vi "test1-testModuleExitEventAPI.vi"(8 "error in (no error)":errorcluster, 11 "TestCase in":refnum<class "testcase-CSMNonCSMCallerSupportAPI.lvclass">) -> (0 "error out":errorcluster, 3 "TestCase out":refnum<class "testcase-CSMNonCSMCallerSupportAPI.lvclass">)   [LabVIEW 2017, in "testcase-CSMNonCSMCallerSupportAPI.lvclass"]
uses:
  testcase-CSMNonCSMCallerSupportAPI.lvclass
  InternalCluster.ctl
  State_Cluster.ctl
  GlobalVariable_CSMModeData.vi
  <vilib>/addons/_JKI Toolkits/VI Tester/TestCase.llb/TestCase.lvclass
  src/user.lib/_NEVSTOP/Communicable State Machine(CSM)/Communicable State Machine.lvlib
  C:/Program Files (x86)/National Instruments/LabVIEW 2017/vi.lib/addons/_JKI Toolkits/VI Tester/TestCase.llb/TestCase.lvclass
panel:
  out "LoopCount":i32
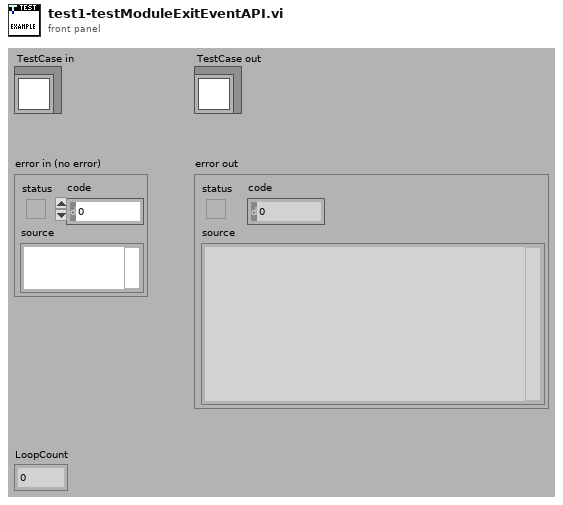
[diagram p1: front panel]
types:
  T1 = typedef "testcase-CSMNonCSMCallerSupportAPI.lvclass/InternalCluster.ctl" = cluster{"Mode":enum16{"Invalid", "Others", "WorkerAgent or Chain"}, "#Nodes":u32}
  T2 = typedef "testcase-CSMNonCSMCallerSupportAPI.lvclass/State_Cluster.ctl" = enum16{"Idle", "Initialize", "PreExit", "Exit"}
  T3 = enum16{"Invalid", "Others", "WorkerAgent or Chain"}
  T4 = typedef "Communicable State Machine.lvlib/_CSM_MODE.ctl" = enum16{"Not Exist", "Stand Alone", "CSM", "Worker", "Worker Agent", "Chain Node", "Chain"}
  T5 = cluster{"Module Exit event occured":bool, "Exit until all nodes exited":bool}
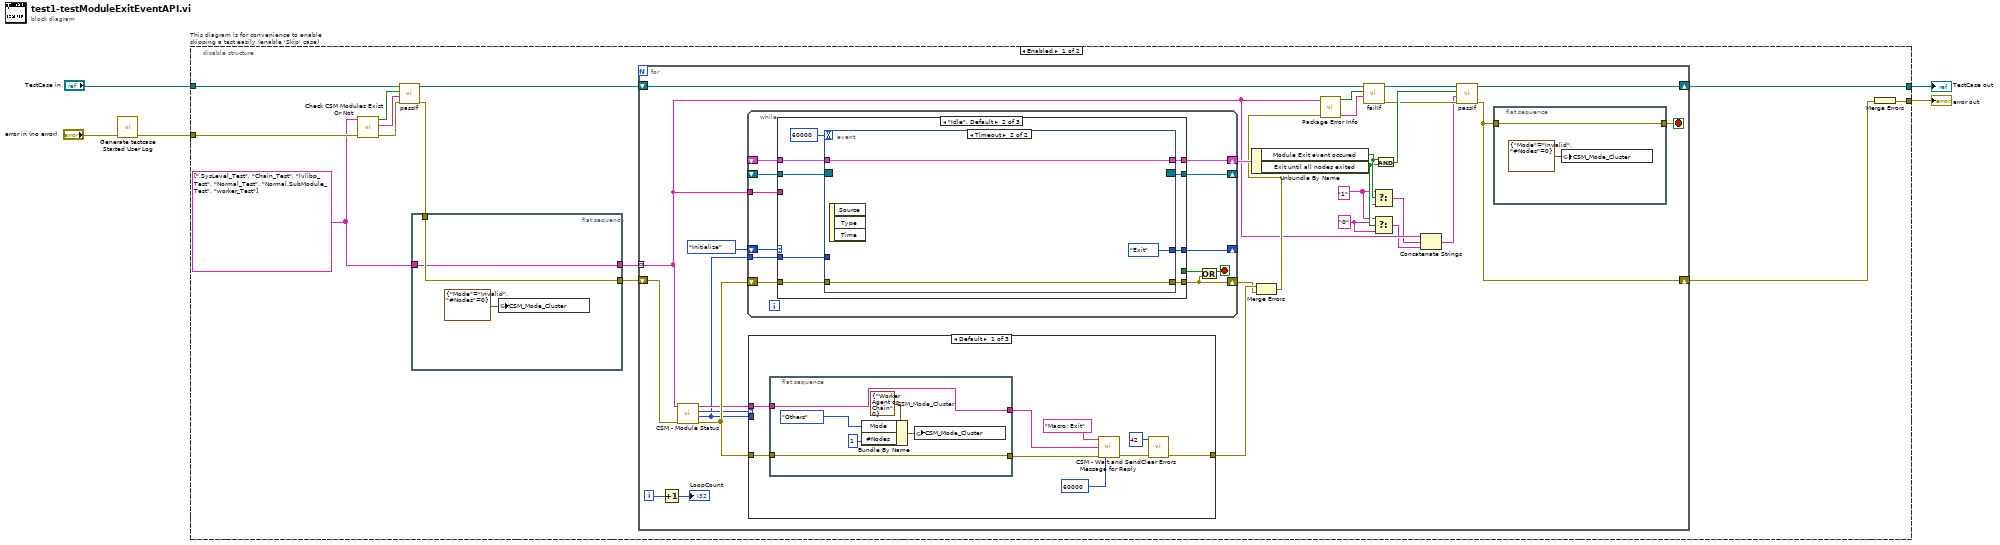
[diagram p0: block diagram]
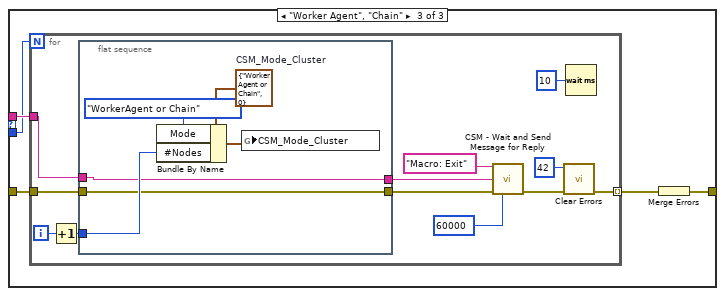
[diagram p3: hidden frame]
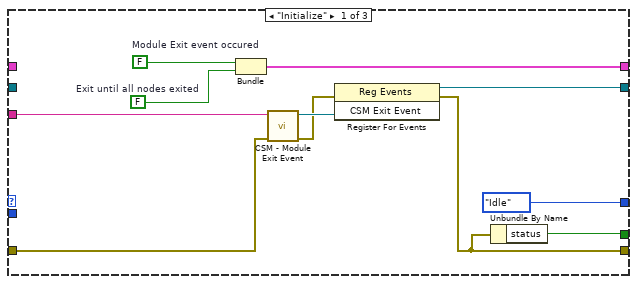
[diagram p4: hidden frame]
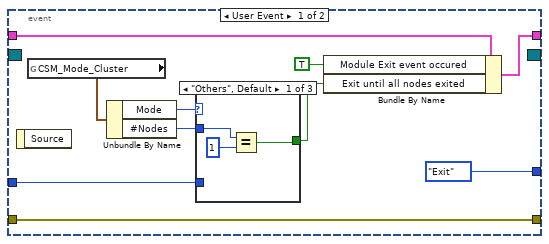
[diagram p5: hidden frame]
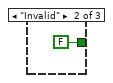
[diagram p6: hidden frame]
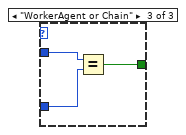
[diagram p7: hidden frame]
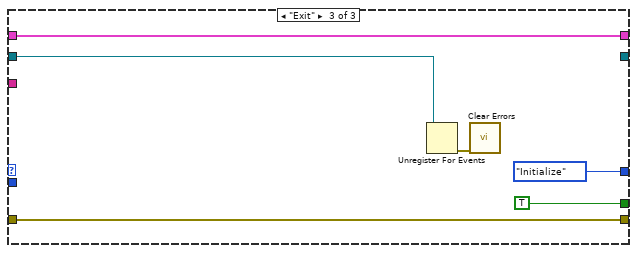
[diagram p8: hidden frame]
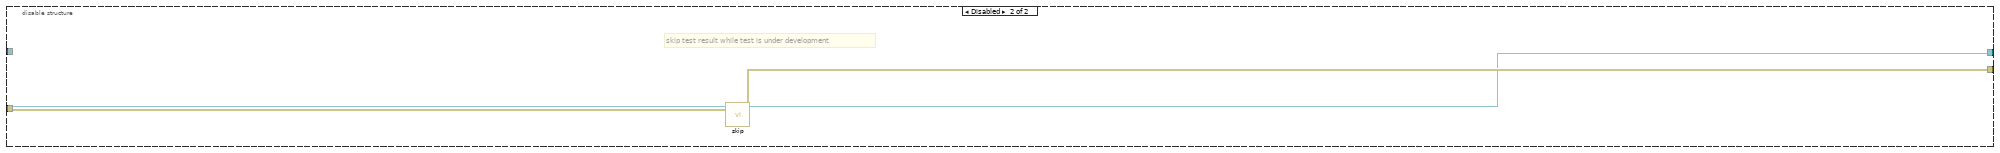
[diagram p9: hidden frame]
diagram:
  n1 = call "Generate testcase Started User Log.vi"("Error In"="error in (no error)") -> ("error out"=w1:errorcluster)  [unwired: 10 in]
  n2 = disable-structure "This diagram is for convenience to enable skipping a test easily (enable 'Skip' case)" shown="Enabled" {
    disable-tunnel: "TestCase in" -> [w11 w153]
    disable-tunnel: [w17 w151] -> w2
    disable-tunnel: [w16 w152] -> w4
    disable-tunnel: w1 -> [w9 w150]
    frame Enabled {
      w6 = string[] [".SysLevel_Test", "Chain_Test", "lvlibp_Test", "Normal_Test", "Normal.SubModule_Test", "worker_Test"] ("Module Names in All Scope")
      n3 = call "Check CSM Modules Exist Or Not.vi"("error in"=w9, "CSM names in"=w6) -> ("error out"=w12:errorcluster, "Debug string"=w13:string, "All Modules Exist?"=w14:bool)  [unwired: 7 in]
      n4 = call-dynamic "passIf.vi"("error in (no error)"=w12, "message (\"\")"=w13, "pass"=w14, "TestCase in"=w11) -> ("error out"=w8:errorcluster, "TestCase out"=w10:refnum<class "testcase-CSMNonCSMCallerSupportAPI.lvclass">)  [unwired: 6 in]
      n5 = flat-sequence {
        tunnel: [w20] -> w18
        tunnel: [w19] -> w15
        tunnel: w8 -> [w20]
        tunnel: w6 -> [w19]
        frame #0 {
          n6 = global write "GlobalVariable_CSMModeData.vi" "CSM_Mode_Cluster"(T1 {"Mode"=enum."Invalid", "#Nodes"=0} ("CSM_Mode_Cluster")) -> ()
        }
      }
      n7 = for {
        shift-right: [w31] -> w7
        shift-left: w18 -> [w45]
        shift-right: [w38] -> w17
        shift-left: w10 -> [w35]
        tunnel: w15 -> [w26] mode=indexing
        i -> [w49]
        stop <- w39 stop-if-true
        w27 = "0"
        w28 = "1"
        n8 = Increment(x=w49) -> (x+1=→"LoopCount":i32)
        n9 = call "CSM - Module Status.vi"("Error In"=w45, "CSM Name"=w26) -> ("error out"=w43:errorcluster, "#Nodes"=w40:i32, "Mode"=w42:T4, "CSM Name (Dup)"=w41:string)  [unwired: 5 in, 1 out]
        n10 = while {
          shift-right: [w99] -> _
          shift-left: State_Cluster."Initialize" -> [w97]
          shift-right: [w102] -> _
          shift-left: _ -> [w101]
          shift-right: [w100] -> w47
          shift-left: _ -> [w98]
          shift-right: [w92] -> w22
          shift-left: w43 -> [w95]
          tunnel: w40 -> [w96]
          tunnel: w26 -> [w94]
          stop <- w93 stop-if-true
          n11 = case shown="\"Idle\", Default" w97 {
            tunnel: [w111 _ TRUE] -> w103
            tunnel: [w113 w122 _] -> w102
            tunnel: w101 -> [_ w123 w149]
            tunnel: [w106 w120 w147] -> w100
            tunnel: w98 -> [_ w121 w147]
            tunnel: w95 -> [w112 w117 w145]
            tunnel: [w109 w116 w145] -> w92
            tunnel: [State_Cluster."Idle" w118 State_Cluster."Initialize"] -> w99
            tunnel: w96 -> [_ w115 _]
            tunnel: w94 -> [w104 _ _]
            frame "Initialize" {
              w105 = FALSE  # Exit until all nodes exited
              w107 = FALSE  # Module Exit event occured
              n12 = Bundle("Module Exit event occured"=w107, "Exit until all nodes exited"=w105) -> (w106:T5)  [unwired: 1 in]
              n13 = call "CSM - Module Exit Event.vi"("Error In"=w112, "Name (\"\" to Use UUID) In"=w104) -> ("error out"=w110:errorcluster, "CSM Exit Event"=w114:refnum<user-event>)  [unwired: 7 in, 1 out]
              n14 = register-events(error in=w110, w114) -> (reference out=w113:refnum<event-registration>, error out=w109:errorcluster)  [unwired: 1 in]
              n15 = Unbundle By Name(w109) -> ("status"=w111:bool)
            }
            frame "Idle", Default {
              n16 = event shown="[1] Timeout" {
                selector: w123 -> [_ _]
                dyn-events: [_ _] -> w122
                timeout: 60000 -> [_ _]
                tunnel: [State_Cluster."Exit" State_Cluster."Exit"] -> w118
                tunnel: w121 -> [w132 w143]
                tunnel: [w125 w143] -> w120
                tunnel: w117 -> [w130 w141]
                tunnel: [w130 w141] -> w116
                tunnel: w115 -> [w126 _]
                event User Event {
                  n17 = event-data() -> ()  [unwired: 1 in, 1 out]
                  n18 = global read "GlobalVariable_CSMModeData.vi" "CSM_Mode_Cluster"() -> (w129:T1)
                  n19 = Unbundle By Name(w129) -> ("Mode"=w128:T3, "#Nodes"=w127:u32)
                  n20 = case shown="\"Others\", Default" w128 {
                    tunnel: [w134 FALSE w138] -> w124
                    tunnel: w127 -> [w136 _ w140]
                    tunnel: w126 -> [_ _ w139]
                    frame "Others", Default {
                      n21 = Equal?(x=w136, y=u32 1) -> (x = y?=w134:bool)
                    }
                    frame "Invalid" {
                    }
                    frame "WorkerAgent or Chain" {
                      n22 = Equal?(x=w140, y=w139) -> (x = y?=w138:bool)
                    }
                  }
                  n23 = Bundle By Name(cluster=w132, "Module Exit event occured"=TRUE, "Exit until all nodes exited"=w124) -> (w125:T5)
                }
                event Timeout {
                  n24 = event-data() -> ()  [unwired: 1 in, 3 out]
                }
              }
            }
            frame "Exit" {
              n25 = Unregister For Events(event registration refnum=w149) -> (error out=w148:errorcluster)  [unwired: 1 in]
              n26 = call <vilib>:"Clear Errors.vi"("error in (no error)"=w148) -> ()  [unwired: 5 in, 2 out]
            }
          }
          n27 = Or(x=w103, y=w92) -> (x .or. y?=w93:bool)
        }
        n28 = case shown="Default" w42 {
          tunnel: w43 -> [w55 w68 w73]
          tunnel: w40 -> [_ _ w71]
          tunnel: w41 -> [w57 _ w72]
          tunnel: [w59 w68 w69] -> w44
          frame Default {
            n29 = flat-sequence {
              tunnel: w57 -> [w63]
              tunnel: [w63] -> w56
              tunnel: w55 -> [w62]
              tunnel: [w62] -> w54
              frame #0 {
                w67 = T1 {"Mode"=enum."WorkerAgent or Chain", "#Nodes"=0}  # CSM_Mode_Cluster
                n30 = Bundle By Name(cluster=w67, "Mode"=T3."Others", "#Nodes"=u32 1) -> (w66:T1)
                n31 = global write "GlobalVariable_CSMModeData.vi" "CSM_Mode_Cluster"(w66) -> ()
              }
            }
            n32 = call "CSM - Wait and Send Message for Reply.vi"("State"="Macro: Exit", "Target Module"=w56, "Error In (No Error)"=w54, "Response Timeout (-2 Using Global Settings)"=60000) -> ("error out"=w60:errorcluster)  [unwired: 8 in, 3 out]
            n33 = call <vilib>:"Clear Errors.vi"("error in (no error)"=w60, "specific error code to clear (0: all)"=42) -> ("error out"=w59:errorcluster)  [unwired: 4 in, 1 out]
          }
          frame "Not Exist" {
          }
          frame "Worker Agent", "Chain" {
            n34 = for {
              N: w71 -> [_]
              tunnel: w72 -> [w78]
              tunnel: w73 -> [w76]
              tunnel: [w81] -> w70 mode=indexing
              i -> [w84]
              n35 = Increment(x=w84) -> (x+1=w83:i32)
              n36 = flat-sequence {
                tunnel: w83 -> [w89]
                tunnel: w78 -> [w87]
                tunnel: [w87] -> w77
                tunnel: w76 -> [w86]
                tunnel: [w86] -> w75
                frame #0 {
                  w91 = T1 {"Mode"=enum."WorkerAgent or Chain", "#Nodes"=0}  # CSM_Mode_Cluster
                  n37 = Bundle By Name(cluster=w91, "Mode"=T3."WorkerAgent or Chain", "#Nodes"=w89) -> (w90:T1)
                  n38 = global write "GlobalVariable_CSMModeData.vi" "CSM_Mode_Cluster"(w90) -> ()
                }
              }
              n39 = call "CSM - Wait and Send Message for Reply.vi"("State"="Macro: Exit", "Target Module"=w77, "Error In (No Error)"=w75, "Response Timeout (-2 Using Global Settings)"=60000) -> ("error out"=w82:errorcluster)  [unwired: 8 in, 3 out]
              n40 = call <vilib>:"Clear Errors.vi"("error in (no error)"=w82, "specific error code to clear (0: all)"=42) -> ("error out"=w81:errorcluster)  [unwired: 4 in, 1 out]
              n41 = Wait (ms)(milliseconds to wait=u32 10) -> ()  [unwired: 1 out]
            }
            n42 = Merge Errors(w70) -> (w69:errorcluster)
          }
        }
        n43 = Unbundle By Name(w47) -> ("Module Exit event occured"=w30:bool, "Exit until all nodes exited"=w29:bool)
        n44 = Merge Errors(w44, w22) -> (w32:errorcluster)
        n45 = call "Package Error Info.vi"("error in"=w32, "String in"=w26) -> ("packed error info out"=w36:string, "error status"=w37:bool)  [unwired: 8 in]
        n46 = call-dynamic "failIf.vi"("message (\"\")"=w36, "fail"=w37, "TestCase in"=w35) -> ("error out"=w33:errorcluster, "TestCase out"=w34:refnum<class "testcase-CSMNonCSMCallerSupportAPI.lvclass">)  [unwired: 7 in]
        n47 = Select(t=w28, s=w30, f=w27) -> (s? t:f=w25:string)
        n48 = Select(t=w28, s=w29, f=w27) -> (s? t:f=w24:string)
        n49 = And(x=w30, y=w29) -> (x .and. y?=w46:bool)
        n50 = Concatenate Strings(w26, w25, w24) -> (w23:string)
        n51 = call-dynamic "passIf.vi"("error in (no error)"=w33, "message (\"\")"=w23, "pass"=w46, "TestCase in"=w34) -> ("error out"=w31:errorcluster, "TestCase out"=w38:refnum<class "testcase-CSMNonCSMCallerSupportAPI.lvclass">)  [unwired: 6 in]
        n52 = flat-sequence {
          tunnel: w31 -> [w51]
          tunnel: [w51] -> w39
          frame #0 {
            n53 = global write "GlobalVariable_CSMModeData.vi" "CSM_Mode_Cluster"(T1 {"Mode"=enum."Invalid", "#Nodes"=0} ("CSM_Mode_Cluster")) -> ()
          }
        }
      }
      n54 = Merge Errors(w7) -> (w16:errorcluster)
    }
    frame Disabled {
      # "skip test result while test is under development"
      n55 = call <vilib>:"skip.vi"("error in (no error)"=w150, "TestCase in"=w153) -> ("error out"=w152:errorcluster, "TestCase out"=w151:refnum<class "testcase-CSMNonCSMCallerSupportAPI.lvclass">)  [unwired: 8 in]
    }
  }
  "error out" <- w4
  "TestCase out" <- w2
